vi "Initialize Global1.vi"(0 "System no.":i32=1 min=1 step=1, 5 "error in":errorcluster) -> (19 "error out":errorcluster)   [LabVIEW 2020]
doc: "This VI initializes Global1 according to the given System no."
uses:
  Global1.vi
panel:
  # "This vi initializes Global 1\naccording to the given system no."
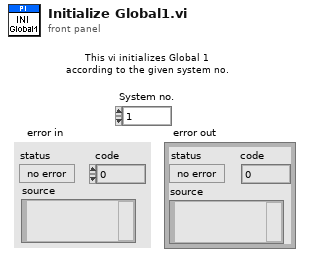
[diagram p1: front panel]
types:
  T1 = cluster{"Host address/name":string, "Port":i32, "Board":i32}[]
  T2 = typedef "Available DLLs.ctl" = u16
  T3 = typedef "Available DLL interfaces.ctl" = u16
  T4 = cluster{"DLL for Device":T2, "DLL Interface":T3, "Parameter":string}[]
  T5 = typedef "Available interfaces.ctl" = u16
  T6 = cluster{"RS232 Portnumber":i32, "Timeout":i32, "RS232 Baud rate":u32, "Interface":T5, "GPIB Bus":i32, "GPIB Address":i32, "GPIB Mode":i32}[]
  T7 = typedef "Termination character.ctl" = enum16{"LF", "CR", "LFCR", "CRLF"}
  T8 = cluster{"data bits":u16, "stop bits":enum16{"1 bit", "1.5 bits", "2 bits"}, "parity":enum16{"no parity", "odd parity", "even parity", "mark parity", "space parity"}}[]
  T9 = cluster{"input XON/XOFF":bool, "input HW Handshake":bool, "input alt HW HShk":bool, "output XON/XOFF":bool, "output HW Handshake":bool, "output alt HW HShk":bool, "XOFF byte ":u8, "XON byte":u8, "parity error byte":u16}[]
  T10 = typedef "Syntax.ctl" = enum16{"GCS 1.0", "GCS 2.0", "GCS 3.0"}
  T11 = cluster{"DLL for Device":T2, "DLL Interface":T3, "Parameter":string}
  T12 = cluster{"RS232 Portnumber":i32, "Timeout":i32, "RS232 Baud rate":u32, "Interface":T5, "GPIB Bus":i32, "GPIB Address":i32, "GPIB Mode":i32}
  T13 = cluster{"input XON/XOFF":bool, "input HW Handshake":bool, "input alt HW HShk":bool, "output XON/XOFF":bool, "output HW Handshake":bool, "output alt HW HShk":bool, "XOFF byte ":u8, "XON byte":u8, "parity error byte":u16}
  T14 = cluster{"data bits":u16, "stop bits":enum16{"1 bit", "1.5 bits", "2 bits"}, "parity":enum16{"no parity", "odd parity", "even parity", "mark parity", "space parity"}}
  T15 = cluster{"Host address/name":string, "Port":i32, "Board":i32}
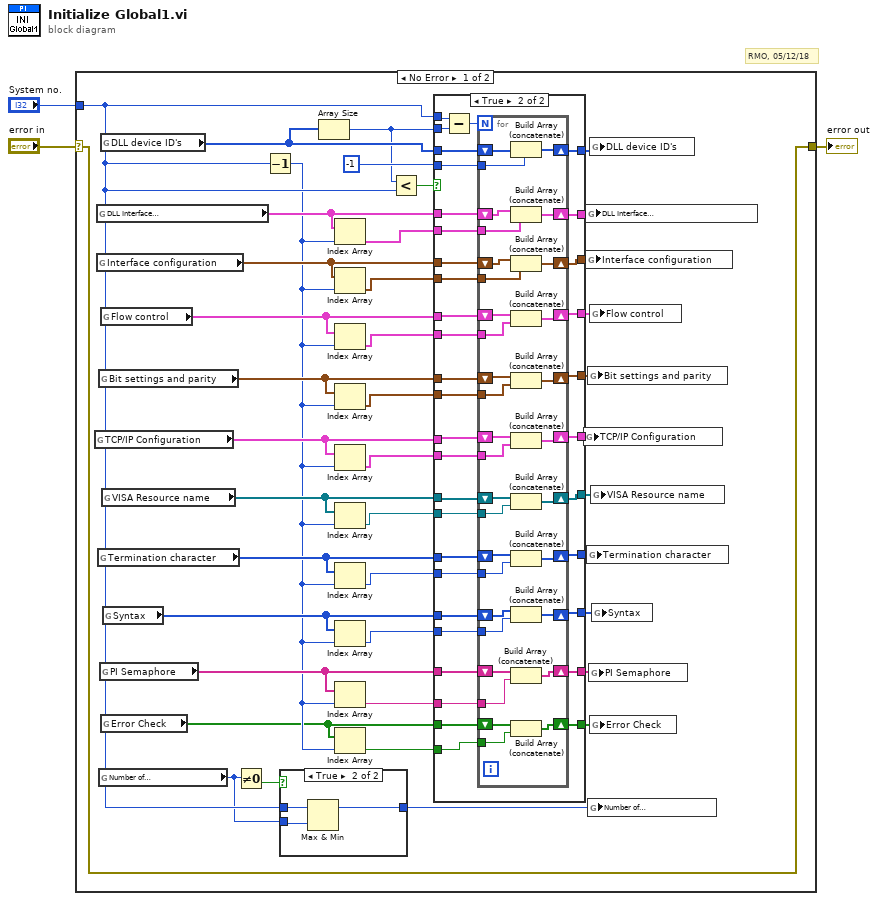
[diagram p0: block diagram]
diagram:
  # "RMO, 05/12/18"
  n1 = case shown="No Error" "error in" {
    selector: "error in" -> [w42 w129]
    tunnel: "System no." -> [w14 _]
    tunnel: [w42 w129] -> w1
    frame No Error {
      n2 = global read "Global1.vi" "TCP/IP Configuration"() -> (w31:T1)
      n3 = global read "Global1.vi" "DLL Interface\nConfiguration"() -> (w39:T4)
      n4 = global read "Global1.vi" "Interface configuration"() -> (w36:T6)
      n5 = global read "Global1.vi" "Termination character"() -> (w29:T7[])
      n6 = global read "Global1.vi" "Bit settings and parity"() -> (w32:T8)
      n7 = global read "Global1.vi" "Number of\nsystems"() -> (w13:i32)
      n8 = global read "Global1.vi" "PI Semaphore"() -> (w10:string[])
      n9 = global read "Global1.vi" "DLL device ID's"() -> (w41:i32[])
      n10 = global read "Global1.vi" "Flow control"() -> (w33:T9)
      n11 = global read "Global1.vi" "Error Check"() -> (w7:bool[])
      n12 = global read "Global1.vi" "VISA Resource name"() -> (w30:refnum<visa-resource-name>[])
      n13 = global read "Global1.vi" "Syntax"() -> (w28:T10[])
      n14 = Not Equal To 0?(x=w13) -> (x != 0?=w15:bool)
      n15 = Decrement(x=w14) -> (x-1=w8:i32)
      n16 = case shown="True" w15 {
        tunnel: w14 -> [w45 w48]
        tunnel: w13 -> [_ w47]
        tunnel: [w45 w46] -> w12
        frame False {
        }
        frame True {
          n17 = Max & Min(x=w48, y=w47) -> (max(x,y)=w46:i32)  [unwired: 1 out]
        }
      }
      n18 = Array Size(array=w41) -> (size(s)=w11:i32)
      n19 = Index Array(array=w39, index=w8) -> (element=w37:T11)
      n20 = Index Array(array=w36, index=w8) -> (element=w34:T12)
      n21 = Index Array(array=w33, index=w8) -> (element=w27:T13)
      n22 = Index Array(array=w32, index=w8) -> (element=w26:T14)
      n23 = Index Array(array=w31, index=w8) -> (element=w25:T15)
      n24 = Index Array(array=w30, index=w8) -> (element=w24:refnum<visa-resource-name>)
      n25 = Index Array(array=w29, index=w8) -> (element=w23:T7)
      n26 = Index Array(array=w28, index=w8) -> (element=w22:T10)
      n27 = Index Array(array=w10, index=w8) -> (element=w9:string)
      n28 = Index Array(array=w7, index=w8) -> (element=w6:bool)
      n29 = Less?(x=w11, y=w14) -> (x < y?=w44:bool)
      n30 = case shown="True" w44 {
        tunnel: w14 -> [_ w94]
        tunnel: w11 -> [_ w93]
        tunnel: w41 -> [w59 w92]
        tunnel: -1 ("error code") -> [_ w91]
        tunnel: [w59 w90] -> w40
        tunnel: w39 -> [w58 w89]
        tunnel: [w58 w88] -> w38
        tunnel: w37 -> [_ w87]
        tunnel: w36 -> [w57 w86]
        tunnel: [w57 w85] -> w35
        tunnel: w34 -> [_ w84]
        tunnel: w33 -> [w56 w83]
        tunnel: w32 -> [w55 w82]
        tunnel: w31 -> [w54 w81]
        tunnel: w30 -> [w53 w80]
        tunnel: w29 -> [w52 w79]
        tunnel: w28 -> [w51 w78]
        tunnel: w27 -> [_ w71]
        tunnel: w26 -> [_ w70]
        tunnel: w25 -> [_ w69]
        tunnel: w24 -> [_ w68]
        tunnel: w23 -> [_ w67]
        tunnel: w22 -> [_ w66]
        tunnel: [w56 w77] -> w21
        tunnel: [w55 w76] -> w20
        tunnel: [w54 w75] -> w19
        tunnel: [w53 w74] -> w18
        tunnel: [w52 w73] -> w17
        tunnel: [w51 w72] -> w16
        tunnel: w10 -> [w50 w65]
        tunnel: w9 -> [_ w64]
        tunnel: w7 -> [w49 w63]
        tunnel: w6 -> [_ w62]
        tunnel: [w50 w61] -> w5
        tunnel: [w49 w60] -> w4
        frame False {
        }
        frame True {
          n31 = Subtract(x=w94, y=w93) -> (x-y=w95:i32)
          n32 = for {
            N: w95 -> [_]
            shift-right: [w128] -> w90
            shift-left: w92 -> [w127]
            tunnel: w91 -> [w126]
            shift-right: [w125] -> w88
            shift-left: w89 -> [w124]
            tunnel: w87 -> [w123]
            shift-right: [w121] -> w85
            shift-left: w86 -> [w122]
            tunnel: w84 -> [w120]
            shift-right: [w113] -> w77
            shift-left: w83 -> [w119]
            shift-right: [w112] -> w76
            shift-left: w82 -> [w118]
            shift-right: [w111] -> w75
            shift-left: w81 -> [w117]
            shift-right: [w110] -> w74
            shift-left: w80 -> [w116]
            shift-right: [w109] -> w73
            shift-left: w79 -> [w115]
            shift-right: [w108] -> w72
            shift-left: w78 -> [w114]
            tunnel: w71 -> [w107]
            tunnel: w70 -> [w106]
            tunnel: w69 -> [w105]
            tunnel: w68 -> [w104]
            tunnel: w67 -> [w103]
            tunnel: w66 -> [w102]
            shift-right: [w100] -> w61
            shift-left: w65 -> [w101]
            tunnel: w64 -> [w99]
            shift-right: [w96] -> w60
            shift-left: w63 -> [w98]
            tunnel: w62 -> [w97]
            n33 = Build Array (concatenate)(w127, w126) -> (w128:i32[])
            n34 = Build Array (concatenate)(w124, w123) -> (w125:T4)
            n35 = Build Array (concatenate)(w122, w120) -> (w121:T6)
            n36 = Build Array (concatenate)(w119, w107) -> (w113:T9)
            n37 = Build Array (concatenate)(w118, w106) -> (w112:T8)
            n38 = Build Array (concatenate)(w117, w105) -> (w111:T1)
            n39 = Build Array (concatenate)(w116, w104) -> (w110:refnum<visa-resource-name>[])
            n40 = Build Array (concatenate)(w115, w103) -> (w109:T7[])
            n41 = Build Array (concatenate)(w114, w102) -> (w108:T10[])
            n42 = Build Array (concatenate)(w101, w99) -> (w100:string[])
            n43 = Build Array (concatenate)(w98, w97) -> (w96:bool[])
          }
        }
      }
      n44 = global write "Global1.vi" "TCP/IP Configuration"(w19) -> ()
      n45 = global write "Global1.vi" "DLL Interface\nConfiguration"(w38) -> ()
      n46 = global write "Global1.vi" "Interface configuration"(w35) -> ()
      n47 = global write "Global1.vi" "Termination character"(w17) -> ()
      n48 = global write "Global1.vi" "Bit settings and parity"(w20) -> ()
      n49 = global write "Global1.vi" "Number of\nsystems"(w12) -> ()
      n50 = global write "Global1.vi" "PI Semaphore"(w5) -> ()
      n51 = global write "Global1.vi" "DLL device ID's"(w40) -> ()
      n52 = global write "Global1.vi" "Flow control"(w21) -> ()
      n53 = global write "Global1.vi" "Error Check"(w4) -> ()
      n54 = global write "Global1.vi" "VISA Resource name"(w18) -> ()
      n55 = global write "Global1.vi" "Syntax"(w16) -> ()
    }
    frame Error {
    }
  }
  "error out" <- w1
